vi "item button.vi"(0 "item array":u32[](array[numeric]), 2 "button":bool[](array[boolean])) -> (7 "confirm":bool[](array[boolean]), 8 "item picture":u32[](array[ring]))   [LabVIEW 2025]
panel:
  out "Numeric":i32
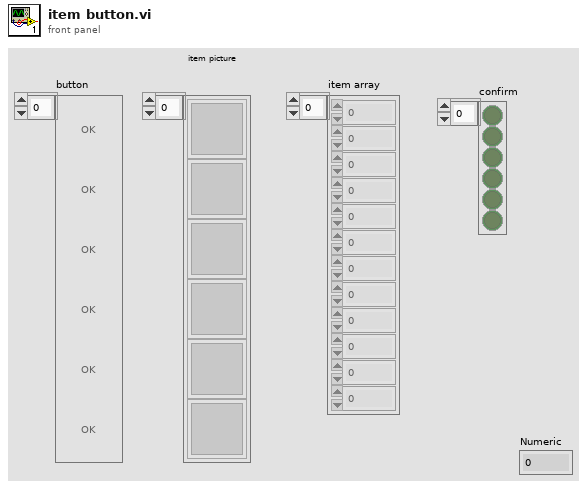
[diagram p1: front panel]
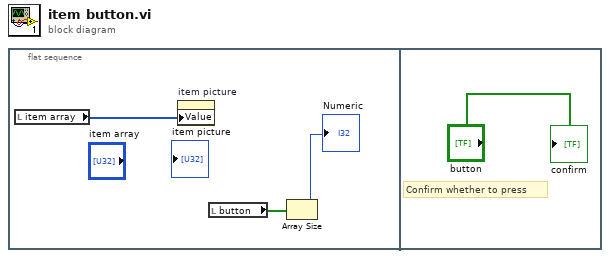
[diagram p0: block diagram]
diagram:
  n1 = flat-sequence {
    frame #0 {
      n2 = local read "item array"() -> (w3:u32[])
      n3 = property on="item picture" class="Arr (strict)"("Value"=w3) -> ()  [unwired: 2 in, 2 out]
      n4 = local read "button"() -> (w2:bool[])
      n5 = Array Size(array=w2) -> (size(s)=→"Numeric":i32)
    }
    frame #1 {
      # "Confirm whether to press"
      "confirm" <- "button"
    }
  }
